vi "6FFT子程序.vi"(4 "window":T2=1 caption="窗" items=["矩形"=0, "Hanning"=1, "Hamming"=2, "Blackman-Harris"=3, "Exact Blackman"=4, "Blackman"=5, "Flat Top"=6, "4阶Blackman-Harris "=7, "7阶Blackman-Harris"=8, "Low Sidelobe"=9, "Blackman Nuttall"=11, "三角"=30, "Bartlett-Hanning"=31, "Bohman"=32, "Parzen"=33, "Welch"=34, "Kaiser"=60, "Dolph-Chebyshev"=61, "高斯"=62], 6 "averaging parameters":T1={"averaging mode"=enum."No averaging", "weighting mode"=enum."Exponential", "number of averages"=10}, 7 "time signal":waveform(dbl) caption="时间信号") -> (0 "幅度":cluster{"f0":dbl, "df":dbl, "magnitude":dbl[]}(graph), 1 "频率的幅度（均方根值）":dbl, 2 "相位":cluster{"f0":dbl, "df":dbl, "phase":dbl[]}(graph), 3 "频率":dbl)   [LabVIEW 2017]
uses:
  <vilib>/Analysis/4window.llb/windowTd.ctl
  <vilib>/measure/maspectr.llb/FFT Spectrum (Mag-Phase) for 1 Chan.vi
  <vilib>/measure/NI_MAPro.lvlib
  <vilib>/Analysis/NI_AALPro.lvlib
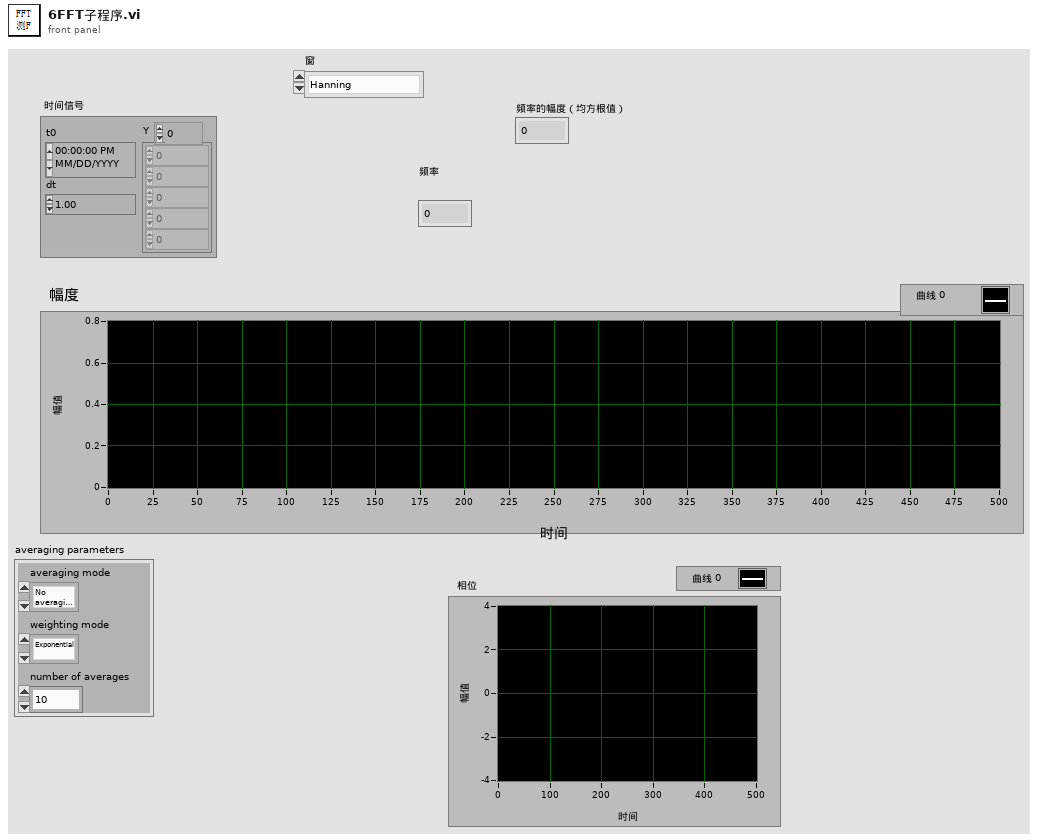
[diagram p1: front panel]
types:
  T1 = cluster{"averaging mode":enum16{"No averaging", "Vector averaging", "RMS averaging", "Peak hold"}, "weighting mode":enum16{"Linear", "Exponential"}, "number of averages":u32}
  T2 = typedef "NI_AALPro.lvlib/windowTd.ctl" = u32
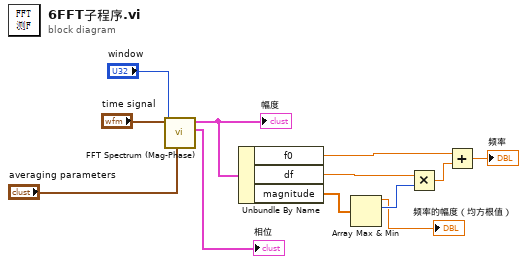
[diagram p0: block diagram]
diagram:
  n1 = call-poly <vilib>:"FFT Spectrum (Mag-Phase).vi"("averaging parameters"="averaging parameters", "window"="window", "time signal"="time signal") -> ("phase"=→"相位":cluster{"f0":dbl, "df":dbl, "phase":dbl[]}, "magnitude"=w12:cluster{"f0":dbl, "df":dbl, "magnitude":dbl[]})  [unwired: 4 in, 3 out]
  "幅度" <- w12
  n2 = Unbundle By Name(w12) -> ("f0"=w10:dbl, "df"=w9:dbl, "magnitude"=w11:dbl[])
  n3 = Array Max & Min(array=w11) -> (max value=→"频率的幅度（均方根值）":dbl, max index (indices)=w8:i32)  [unwired: 2 out]
  n4 = Multiply(x=w9, y=w8) -> (x*y=w7:dbl)
  n5 = Add(x=w10, y=w7) -> (x+y=→"频率":dbl)
